vi "write file header.vi"(8 "error in (no error)":errorcluster, 11 "Log File in":refnum<class "Log File.lvclass">) -> (0 "error out":errorcluster, 3 "Log File out":refnum<class "Log File.lvclass">)   [LabVIEW 2018, in "Log File.lvclass"]
uses:
  Log File.lvclass
  Log File.lvclass/Log File.ctl
panel:
  out "log level":u16(ring) items=[" DEBBUG ", "  INFO  ", "WARNING ", " ERROR  ", "CRITICAL"]
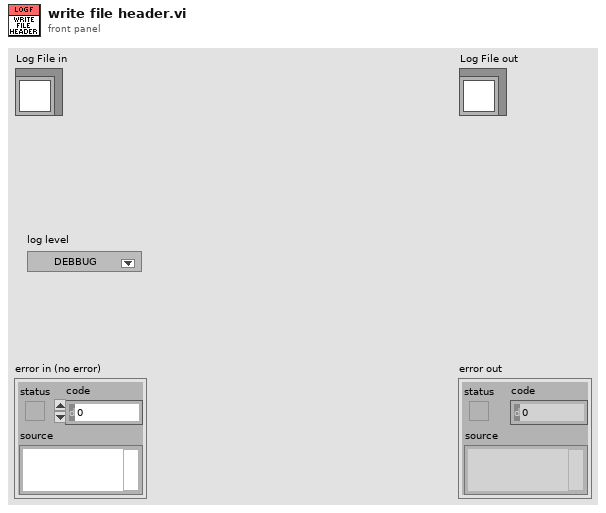
[diagram p1: front panel]
types:
  T1 = typedef "LVDateTimeRec.ctl" = cluster{"fractional second":dbl, "second":i32, "minute":i32, "hour":i32, "day of month":i32, "month":i32, "year":i32, "day of week":i32, "day of year":i32, "DST":i32}
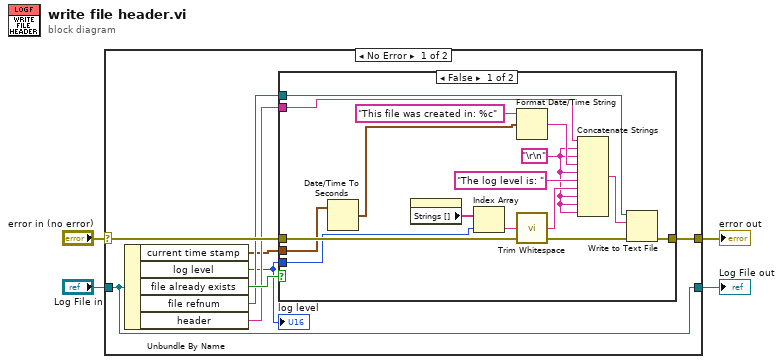
[diagram p0: block diagram]
diagram:
  n1 = case shown="No Error" "error in (no error)" {
    selector: "error in (no error)" -> [w11 w30]
    tunnel: [w12 w30] -> w3
    tunnel: [w10 w29] -> w1
    tunnel: "Log File in" -> [w10 w29]
    frame No Error {
      n2 = Unbundle By Name(w10) -> ("current time stamp"=w6:T1, "log level"=w5:u16, "file already exists"=w9:bool, "file refnum"=w8:refnum<file>, "header"=w7:string)
      "log level" <- w5
      n3 = case shown="False" w9 {
        tunnel: [w27 w28] -> w12
        tunnel: w11 -> [w26 w28]
        tunnel: w8 -> [w24 _]
        tunnel: w7 -> [w23 _]
        tunnel: w6 -> [w22 _]
        tunnel: w5 -> [w17 _]
        frame False {
          w13 = "\r\n"
          n4 = Date/Time To Seconds(2:w22) -> (0:w21:timestamp)  [unwired: 1 in]
          n5 = property on="log level" class="Ring (strict)"() -> ("Strings []"=w18:string[])  [unwired: 2 in, 2 out]
          n6 = Index Array(array=w18, index=w17) -> (element=w16:string)
          n7 = Format Date/Time String(time format string (%c)="This file was created in: %c", seconds (now)=w21) -> (date/time string=w19:string)  [unwired: 1 in]
          n8 = call <vilib>:"Trim Whitespace.vi"("string"=w16) -> ("trimmed string"=w15:string)  [unwired: 1 in]
          n9 = Concatenate Strings(w23, w13, w13, w19, w13, "The log level is: " ("string"), w15, w13, w13, w13) -> (w25:string)
          n10 = Write to Text File(file (use dialog)=w24, text=w25, error in=w26) -> (error out=w27:errorcluster)  [unwired: 1 in, 2 out]
        }
        frame True {
        }
      }
    }
    frame Error {
    }
  }
  "error out" <- w3
  "Log File out" <- w1
